vi "Print Button Pressed.vi"(8 "error in (no error)":errorcluster, 11 "Print Model in":refnum<class "Print Model.lvclass">) -> (0 "error out":errorcluster, 3 "Print Model out":refnum<class "Print Model.lvclass">)   [LabVIEW 2015, in "Print Model.lvlib" / "Print Model.lvclass"]
uses:
  Print Model.lvclass
  <vilib>/Utility/miscctls.llb/LVPositionTypeDef.ctl
  Print Model Messages/Start Print Msg/Start Print Msg.lvclass
  UI Controller/UI Controller Messages/Hide Subpanel Msg/Hide Subpanel Msg.lvclass
  UI Controller/UI Controller Messages/Hide Subpanel Msg/Hide Subpanel Msg.lvclass/Hide Subpanel Msg.ctl
  <vilib>/ActorFramework/Actor/Actor.lvclass/Actor.ctl
  <vilib>/ActorFramework/Message Enqueuer/Message Enqueuer.lvclass/Message Enqueuer.ctl
  <vilib>/ActorFramework/Self-Addressed Msg/Self-Addressed Msg.lvclass/Self-Addressed Msg.ctl
  <vilib>/ActorFrameworkMVC/View Controller/View Controller Messages/Insert Subpanel Msg/Insert Subpanel Msg.lvclass/Insert Subpanel Msg.ctl
  <vilib>/ActorFrameworkMVC/View Controller/View Controller Messages/Move Subpanel Msg/Move Subpanel Msg.lvclass/Move Subpanel Msg.ctl
  <vilib>/ActorFramework/Message Enqueuer/Init from Existing Queue.vi
  <vilib>/ActorFramework/Message Enqueuer/Enqueue.vi
  <vilib>/ActorFramework/Message Priority Queue/Priority Enqueue.vi
  <vilib>/ActorFramework/Message Enqueuer/Message Enqueuer.lvclass
  <vilib>/ActorFramework/Self-Addressed Msg/Self-Addressed Msg.lvclass
  <vilib>/ActorFrameworkMVC/View Controller/View Controller Messages/Insert Subpanel Msg/Insert Subpanel Msg.lvclass
  <vilib>/ActorFrameworkMVC/View Controller/View Controller Messages/Move Subpanel Msg/Move Subpanel Msg.lvclass
  <vilib>/ActorFramework/Actor/Actor.lvclass
panel:
  # "NOTICE -- YOU MUST LEAVE THIS NOTICE IN PLACE.\n\nCopyright (c) 2015, LIANG LIU Shawn.Liu.cn@gmail.com\nAll rights reserved.\n\nRedistribution and use in source and binary forms, with or without modification, are permitted provided that the following conditions are met:\n-Redistributions of source code must retain the above copyright notice, this list of conditions and the following disclaimer.\n-Redistributions in binary form must reproduce the above copyright notice, this list of conditions and the following disclaimer in the documentation and/or other materials provided with the distribution.\n-Neither the name of the eLp nor the names of its contributors may be used to endorse or promote products derived from this software without specific prior written permission.\n\nTHIS SOFTWARE IS PROVIDED BY THE COPYRIGHT HOLDERS AND CONTRIBUTORS \"AS IS\" AND ANY EXPRESS OR IMPLIED WARRANTIES, INCLUDING, BUT NOT LIMITED TO, THE IMPLIED WARRANTIES OF MERCHANTABILITY AND FITNESS FOR A PARTICULAR PURPOSE ARE DISCLAIMED. IN NO EVENT SHALL THE COPYRIGHT HOLDER OR CONTRIBUTORS BE LIABLE FOR ANY DIRECT, INDIRECT, INCIDENTAL, SPECIAL, EXEMPLARY, OR CONSEQUENTIAL DAMAGES (INCLUDING, BUT NOT LIMITED TO, PROCUREMENT OF SUBSTITUTE GOODS OR SERVICES; LOSS OF USE, DATA, OR PROFITS; OR BUSINESS INTERRUPTION) HOWEVER CAUSED AND ON ANY THEORY OF LIABILITY, WHETHER IN CONTRACT, STRICT LIABILITY, OR TORT (INCLUDING NEGLIGENCE OR OTHERWISE) ARISING IN ANY WAY OUT OF THE USE OF THIS SOFTWARE, EVEN IF ADVISED OF THE POSSIBILITY OF SUCH DAMAGE."
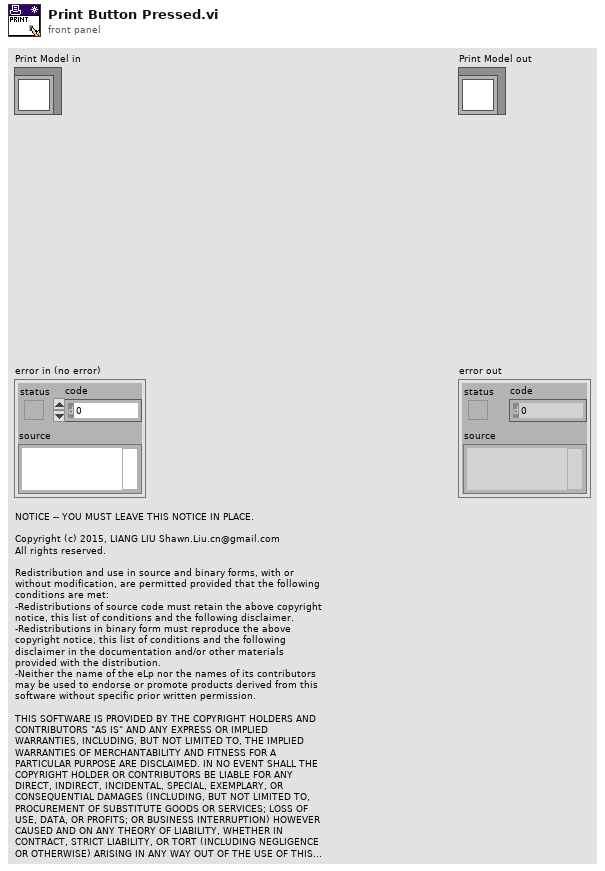
[diagram p1: front panel]
types:
  T1 = typedef "LVPositionTypeDef.ctl" = cluster{"Left":i32, "Top":i32}
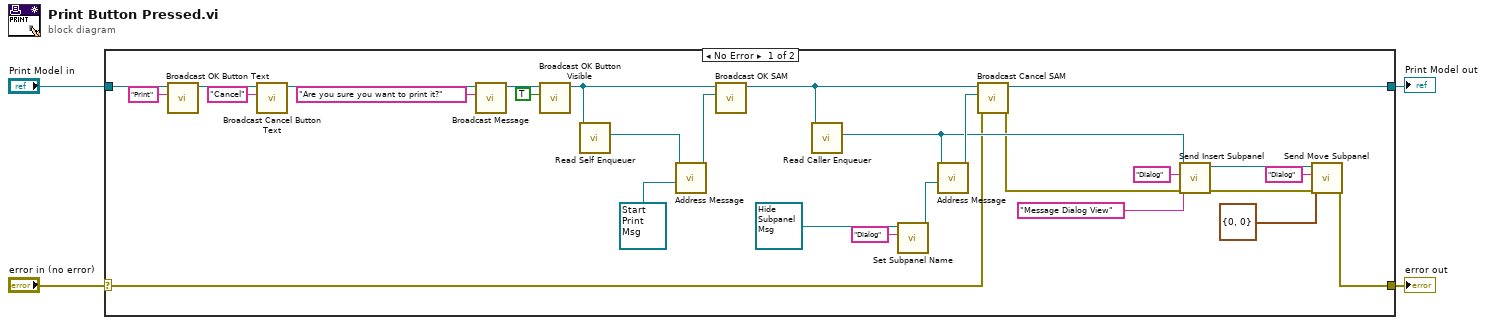
[diagram p0: block diagram]
diagram:
  n1 = case shown="No Error" "error in (no error)" {
    selector: "error in (no error)" -> [w9 w34]
    tunnel: "Print Model in" -> [w30 w33]
    tunnel: [w26 w33] -> w3
    tunnel: [w8 w34] -> w1
    frame No Error {
      n2 = call "Broadcast OK Button Text.vi"("OK Button Text"="Print", "Print Model in"=w30) -> ("Print Model out"=w32:refnum<class "Print Model.lvclass">)  [unwired: 8 in, 1 out]
      n3 = call "Broadcast Cancel Button Text.vi"("Cancel Button Text"="Cancel", "Print Model in"=w32) -> ("Print Model out"=w31:refnum<class "Print Model.lvclass">)  [unwired: 8 in, 1 out]
      n4 = call "Broadcast Message.vi"("Message"="Are you sure you want to print it?", "Print Model in"=w31) -> ("Print Model out"=w15:refnum<class "Print Model.lvclass">)  [unwired: 8 in, 1 out]
      n5 = call "Broadcast OK Button Visible.vi"("OK Button Visible"=TRUE, "Print Model in"=w15) -> ("Print Model out"=w11:refnum<class "Print Model.lvclass">)  [unwired: 8 in, 1 out]
      n6 = call <vilib>:"Read Self Enqueuer.vi"("Actor"=w11) -> ("Self Enqueuer"=w14:refnum<class "Message Enqueuer.lvclass">)  [unwired: 10 in]
      n7 = call <vilib>:"Address Message.vi"("Message"=refnum<class "Start Print Msg.lvclass"> refnum ("Print Model.lvlib:Start Print Msg.lvclass"), "Destination"=w14) -> ("Self-Addressed Message"=w13:refnum<class "Self-Addressed Msg.lvclass">)  [unwired: 9 in]
      n8 = call "Broadcast OK SAM.vi"("OK SAM"=w13, "Print Model in"=w11) -> ("Print Model out"=w16:refnum<class "Print Model.lvclass">)  [unwired: 8 in, 1 out]
      n9 = call <vilib>:"Read Caller Enqueuer.vi"("Actor"=w16) -> ("Caller Enqueuer"=w18:refnum<class "Message Enqueuer.lvclass">)  [unwired: 10 in]
      n10 = call "Set Subpanel Name.vi"("Subpanel Name"="Dialog", "Hide Subpanel Msg in"=refnum<class "Hide Subpanel Msg.lvclass"> refnum ("View Controller.lvlib:Move Subpanel Msg.lvclass")) -> ("Hide Subpanel Msg out"=w5:refnum<class "Hide Subpanel Msg.lvclass">)  [unwired: 9 in]
      n11 = call <vilib>:"Address Message.vi"("Message"=w5, "Destination"=w18) -> ("Self-Addressed Message"=w25:refnum<class "Self-Addressed Msg.lvclass">)  [unwired: 9 in]
      n12 = call "Broadcast Cancel SAM.vi"("error in (no error)"=w9, "Cancel SAM"=w25, "Print Model in"=w16) -> ("error out"=w17:errorcluster, "Print Model out"=w26:refnum<class "Print Model.lvclass">)  [unwired: 7 in]
      n13 = call <vilib>:"Send Insert Subpanel.vi"("error in (no error)"=w17, "View Name"="Message Dialog View" ("Subpanel Name"), "Subpanel Name"="Dialog", "Message Enqueuer"=w18) -> ("error out"=w22:errorcluster, "Message Enqueuer out"=w21:refnum<class "Message Enqueuer.lvclass">)  [unwired: 6 in]
      n14 = call <vilib>:"Send Move Subpanel.vi"("error in (no error)"=w22, "Position"=T1 {"Left"=0, "Top"=0}, "Subpanel Name"="Dialog", "Message Enqueuer"=w21) -> ("error out"=w8:errorcluster)  [unwired: 6 in, 1 out]
    }
    frame Error {
    }
  }
  "error out" <- w1
  "Print Model out" <- w3
